vi "setpointsGlobal.vi"() -> ()   [LabVIEW 2013]
uses:
  setpointCluster.ctl
panel:
  in  "Setpoint Cluster":T1={"Modulus Setpoint"=1.8, "Argument Setpoint"=0.0}
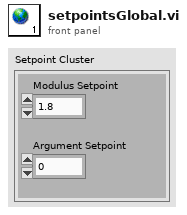
[diagram p1: front panel]
types:
  T1 = typedef "setpointCluster.ctl" = cluster{"Modulus Setpoint":dbl, "Argument Setpoint":dbl}
diagram:
